vi "follow the peak.vi"(0 "omega(0)":dbl, 5 "gamma":dbl, 11 "follow the peak Con":T1={"factor"=3.0, "omega ?"=TRUE, "gamma ?"=TRUE, "max (kHz)"=3.0, "is clean"=TRUE, "acceptance"=0.3, "history - length"=10}, 12 "cursor bracket - data 2":refnum<vi>, 13 "cursor bracket - fragment 2":refnum<vi>) -> (4 "interpolated omega":dbl, 6 "interpolated gamma":dbl, 15 "follow the peak is clean out":bool)   [LabVIEW 2021]
uses:
  cursor window action.ctl
  cursor winow.ctl
  follow the peak control.ctl
panel:
  in  "cursor bracket in":T2={"left"=2044.0881763527054, "right "=2126.7657992565055, "center"=2085.4269878046052, "window"=82.67762290380006, "cursors"=[], "relative"=0, "absolute"=0, "fixed vertical offset"=2421.6740576496672, "vertical offset"=2421.6740576496672, "skew"=2421.6740576496672, "default window frac"=2421.6740576496672, "kind"=enum."fancy", "skew.left"=2.0, "skew.right"=0.0, "Plot ref"=refnum, "wing order"=enum."back"}
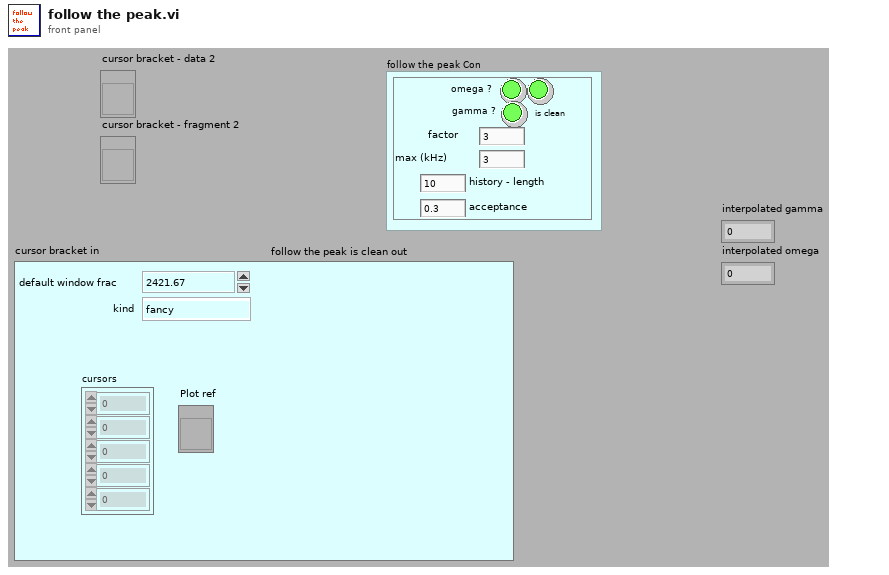
[diagram p1: front panel]
types:
  T1 = typedef "follow the peak control.ctl" = cluster{"factor":dbl, "omega ?":bool, "gamma ?":bool, "max (kHz)":dbl, "is clean":bool, "acceptance":dbl, "history - length":i32}
  T2 = typedef "cursor winow.ctl" = cluster{"left":dbl, "right ":dbl, "center":dbl, "window":dbl, "cursors":i32[], "relative":i32, "absolute":i32, "fixed vertical offset":dbl, "vertical offset":dbl, "skew":dbl, "default window frac":dbl, "kind":enum16{"symmetric", "skewed", "fancy"}, "skew.left":dbl, "skew.right":dbl, "Plot ref":refnum<vi>, "wing order":enum16{"forw", "back"}}
  T3 = typedef "cursor window action.ctl" = enum16{"balance", "h. offset change", "cursor moves", "change center", "change window", "init", "check", "reset", "set y to middle", "idle", "-write all Y", "-write left.X", "-write center.X", "-write right.X", "-write all X", "-change center", "-change window", "-change skew", "-read cursor 2", "-read cursor 1", "-read cursor 0", "-read all cursors", "-reset", "-read plot scale", "-set y to middle", "-Q: center.Y is visible", "-Q: window is visible", "-parse center.Y", "-right left from center", "-left move", "-right move", "-set center.Y", "-empty", "-set cursors to default", "-check", "-write center.Y", "-copy cursor 1", "-copy cursor 0", "-copy cursor 2", "move right", "move left", "shrink", "broaden", "skew up", "skew down", "-write plot scale", "zoom X", "change cen&win", "zoom to all data", "color--red", "color--green", "color--yellow", "read", "zoom out", "zoom in", "slide right", "slide left", "set range aspect ratio to 1", "move to window range", "--move to window range"}
  T4 = cluster{"left":dbl, "right ":dbl, "center":dbl, "window":dbl, "cursors":i32[], "relative":i32, "absolute":i32, "fixed vertical offset":dbl, "vertical offset":dbl, "skew":dbl, "default window frac":dbl, "kind":enum16{"symmetric", "skewed", "fancy"}, "skew.left":dbl, "skew.right":dbl, "Plot ref":refnum<vi>, "wing order":enum16{"forw", "back"}}
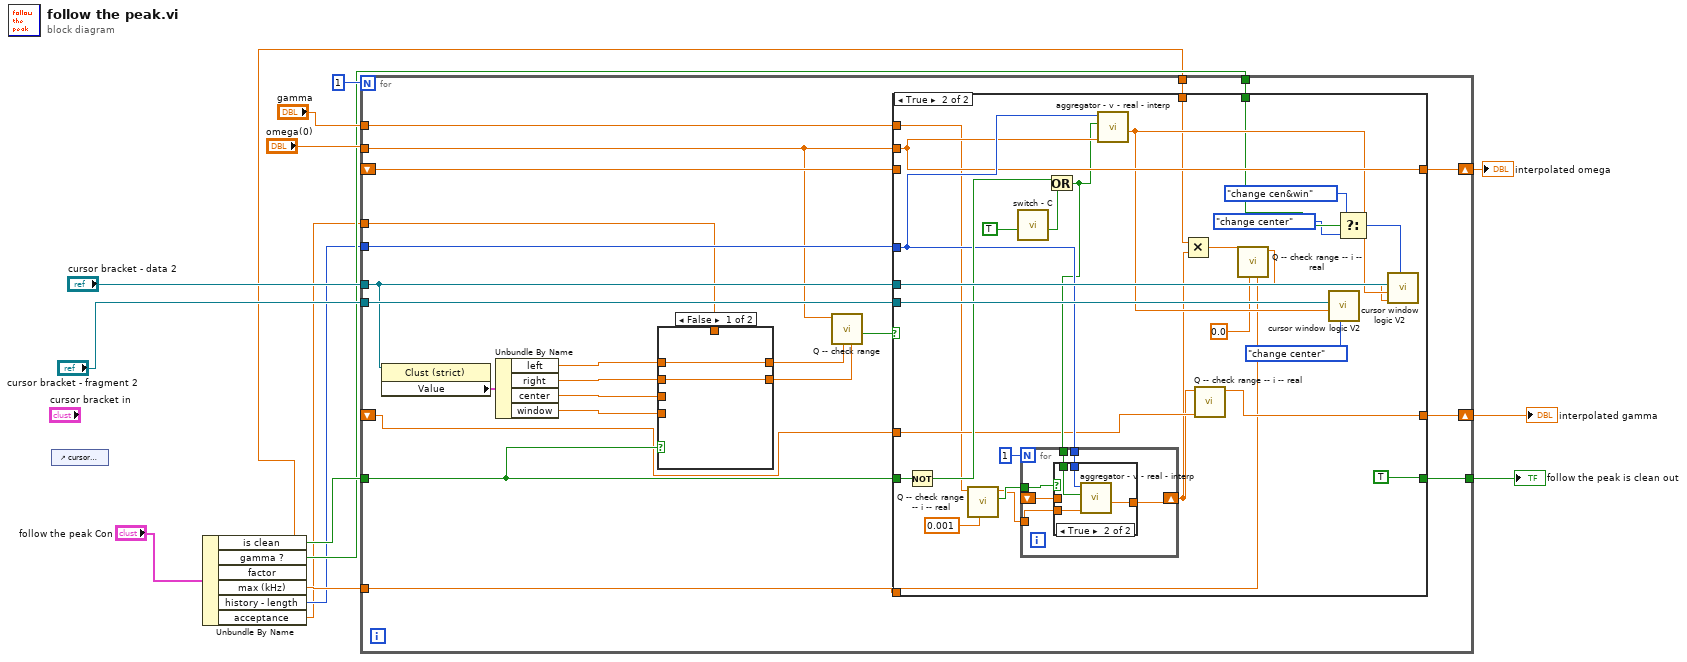
[diagram p0: block diagram]
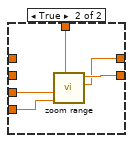
[diagram p2: hidden frame]
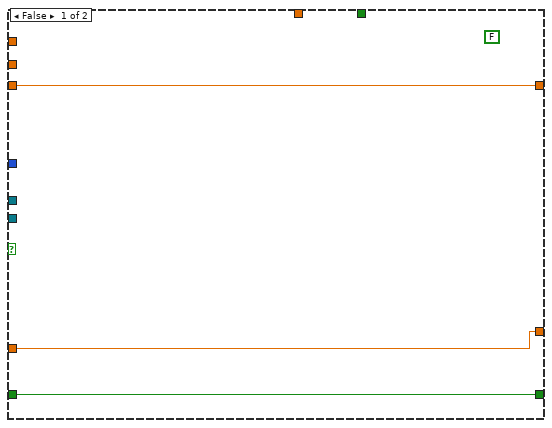
[diagram p3: hidden frame]
diagram:
  n1 = control-ref of="cursor bracket in"() -> ()  [unwired: 1 out]
  n2 = Unbundle By Name("follow the peak Con") -> ("is clean"=w6:bool, "gamma ?"=w5:bool, "factor"=w4:dbl, "max (kHz)"=w3:dbl, "history - length"=w2:i32, "acceptance"=w1:dbl)
  n3 = for {
    N: 1 -> [_]
    tunnel: w2 -> [w38]
    shift-right: [w37] -> w10
    shift-left: _ -> [w36]
    tunnel: "cursor bracket - data 2" -> [w33]
    tunnel: "cursor bracket - fragment 2" -> [w35]
    tunnel: "omega(0)" -> [w31]
    tunnel: w1 -> [w22]
    tunnel: [w30] -> w13
    tunnel: w6 -> [w29]
    tunnel: "gamma" -> [w21]
    shift-right: [w20] -> w11
    shift-left: _ -> [w19]
    tunnel: w4 -> [w18]
    tunnel: w5 -> [w17]
    tunnel: w3 -> [w16]
    n4 = property class="Clust (strict)"(reference=w33) -> ("Value"=w34:T4)  [unwired: 1 in, 2 out]
    n5 = Unbundle By Name(w34) -> ("left"=w24:dbl, "right"=w23:dbl, "center"=w28:dbl, "window"=w27:dbl)
    n6 = case shown="False" w29 {
      tunnel: w28 -> [_ w45]
      tunnel: w27 -> [_ w44]
      tunnel: [w39 w43] -> w26
      tunnel: [w40 w42] -> w25
      tunnel: w24 -> [w40 _]
      tunnel: w23 -> [w39 _]
      tunnel: w22 -> [_ w41]
      frame False {
      }
      frame True {
        n7 = call "zoom range.vi"("factor"=w41, "window"=w44, "center"=w45) -> ("left out"=w42:dbl, "right out"=w43:dbl)  [unwired: 5 in, 2 out]
      }
    }
    n8 = call "Q -- check range.vi"("upper"=w26, "lower"=w25, "number"=w31) -> ("in range?"=w32:bool)  [unwired: 4 in, 4 out]
    n9 = case shown="True" w32 {
      tunnel: w38 -> [_ w69]
      tunnel: [w48 w68] -> w37
      tunnel: w36 -> [w48 _]
      tunnel: w33 -> [_ w75]
      tunnel: w35 -> [_ w74]
      tunnel: w31 -> [_ w68]
      tunnel: [w47 TRUE] -> w30
      tunnel: w29 -> [w47 w72]
      tunnel: w21 -> [_ w63]
      tunnel: [w46 w64] -> w20
      tunnel: w19 -> [w46 w65]
      tunnel: w18 -> [_ w57]
      tunnel: w17 -> [_ w56]
      tunnel: w16 -> [_ w50]
      frame False {
        (unwired) FALSE
      }
      frame True {
        n10 = Not(x=w72) -> (.not. x?=w71:bool)
        n11 = call "Q -- check range -- i -- real.vi"("lower"=0.001, "number"=w63) -> ("in range?"=w61:bool, "number in range"=w60:dbl)  [unwired: 7 in, 1 out]
        n12 = call "switch - C.vi"("switch"=TRUE) -> ("result"=w76:bool)  [unwired: 10 in]
        n13 = Or(x=w71, y=w76) -> (x .or. y?=w67:bool)
        n14 = for {
          N: 1 -> [_]
          tunnel: w69 -> [w83]
          tunnel: w67 -> [w82]
          tunnel: w60 -> [w80]
          shift-right: [w81] -> w58
          shift-left: _ -> [w78]
          tunnel: w61 -> [w79]
          n15 = case shown="True" w79 {
            tunnel: w83 -> [_ w88]
            tunnel: w82 -> [_ w87]
            tunnel: [w84 w86] -> w81
            tunnel: w80 -> [_ w85]
            tunnel: w78 -> [w84 _]
            frame False {
            }
            frame True {
              n16 = call "aggregator - v - real - interp.vi"("number"=w85, "init?"=w87, "requested size"=w88) -> ("interp average"=w86:dbl)  [unwired: 5 in, 3 out]
            }
          }
        }
        n17 = call "aggregator - v - real - interp.vi"("number"=w68, "init?"=w67, "requested size"=w69) -> ("interp average"=w66:dbl)  [unwired: 5 in, 3 out]
        n18 = Multiply(x=w57, y=w58) -> (x*y=w52:dbl)
        n19 = call "Q -- check range -- i -- real.vi"("default"=w65, "number"=w58) -> ("number in range"=w64:dbl)  [unwired: 7 in, 2 out]
        n20 = call "Q -- check range -- i -- real.vi"("upper"=w50, "lower"=0.0, "number"=w52) -> ("number in range"=w49:dbl)  [unwired: 6 in, 2 out]
        n21 = call "cursor window logic V2.vi"("cursor window action"=cursor_window_action."change center", "center"=w66, "cursor window in"=w74) -> ()  [unwired: 7 in, 2 out]
        n22 = Select(t=cursor_window_action."change cen&win" ("cursor window action"), s=w56, f=cursor_window_action."change center" ("cursor window action")) -> (s? t:f=w53:T3)
        n23 = call "cursor window logic V2.vi"("cursor window action"=w53, "window"=w49, "center"=w66, "cursor window in"=w75) -> ()  [unwired: 6 in, 2 out]
      }
    }
  }
  "follow the peak is clean out" <- w13
  "interpolated gamma" <- w11
  "interpolated omega" <- w10
